vi "Terminal-LoadSpectrum-Controller.vi"(8 "error in (no error)":errorcluster caption="错误输入（无错误）", 11 "命令":T1(ring)) -> (0 "error out":errorcluster caption="错误输出")   [LabVIEW 2014]
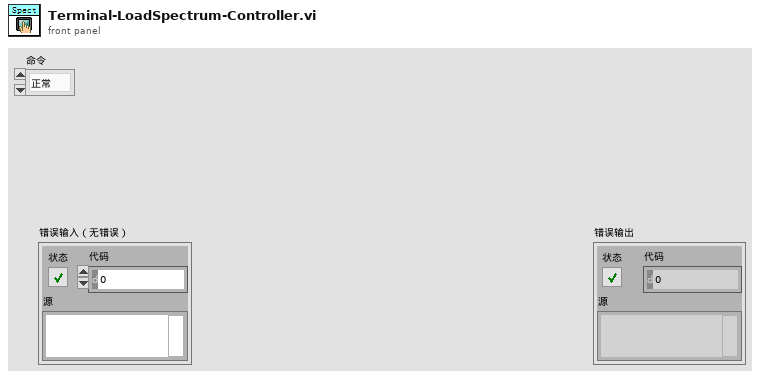
[diagram p1: front panel]
types:
  T1 = enum16{"正常", "内部异常", "修改载荷谱", "外部异常", "外部停止", "其他"}
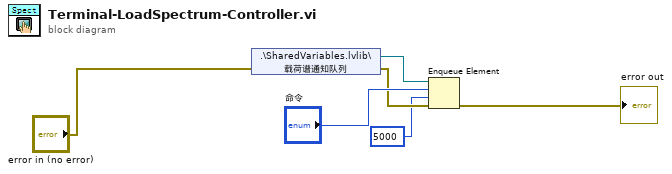
[diagram p0: block diagram]
diagram:
  n1 = shared-variable ".\\SharedVariables.lvlib\\载荷谱通知队列"(error in="error in (no error)") -> (w6:refnum<queue>, error out=w3:errorcluster)
  n2 = Enqueue Element(queue=w6, element="命令", timeout in ms (-1)=5000 ("超时毫秒(-1)"), error in (no error)=w3) -> (error out=→"error out":errorcluster)  [unwired: 2 out]
